vi "averager.vi"() -> ()   [LabVIEW 2015]
uses:
  <vilib>/rvi/IPIntegrationNode/IPINode_Typedef/niFpgaIPINodeSupportedFamilies.ctl
  <vilib>/rvi/Emulation/niFpgaGetClockAttributes.vi
  <vilib>/rvi/Emulation/niFpgaSctlEmulationGetInTimedLoop.vi
  <vilib>/rvi/Emulation/niFpgaEmulationReportErrorSimple.vi
  <vilib>/rvi/IPIntegrationNode/IPINode_Utilities/niFpgaIPINodeSimCore.vi
  <vilib>/rvi/Emulation/niFpgaCriticalErrorInLSC.vi
  <vilib>/rvi/XilinxIP/XIPIN_XNode/niFpgaXIPIN.xnode
  averager/Accumulator/Accumulator_53DC2439CD9149F49F85B82DAD68175F.dll
  <vilib>/rvi/IPIntegrationNode/IPINode_Xnode/niFpgaIPINode.xnode
panel:
  out "Numeric 2":fxp<+/-,32,16>
  out "Numeric":u64
  in  "bypass":bool
  in  "c_in":bool
  in  "Array":fxp<+,32,32>[](array[numeric])
  in  "n":i32
  out "q":bool[](array[boolean])
  in  "sclr":bool
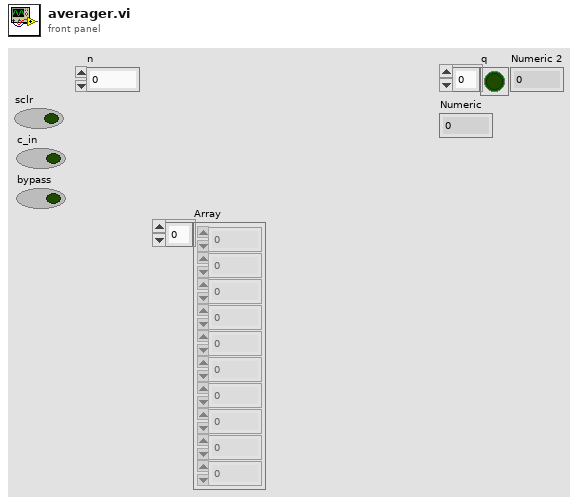
[diagram p1: front panel]
types:
  T1 = typedef "niFpgaIPINodeSupportedFamilies.ctl" = cluster{"unlimited?":bool, "supported targets":string[]}
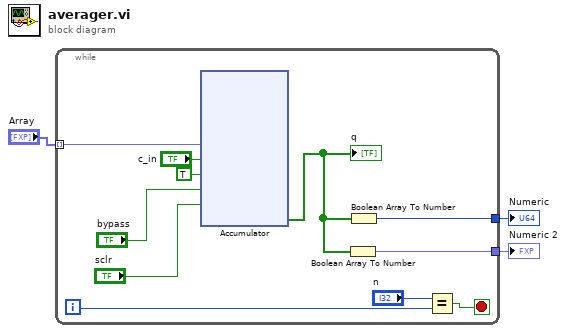
[diagram p0: block diagram]
diagram:
  n1 = while {
    tunnel: "Array" -> [w7] mode=indexing
    tunnel: [w6] -> w1
    tunnel: [w4] -> w2
    i -> [w12]
    stop <- w13 stop-if-true
    n2 = xnode ("Accumulator")("b"=w7, "c_in"="c_in", "ce"=TRUE, "bypass"="bypass", "sclr"="sclr") -> ("q"=w5:bool[])
    "q" <- w5
    n3 = Boolean Array To Number(Boolean array=w5) -> (number=w6:fxp<+/-,32,16>)
    n4 = Boolean Array To Number(Boolean array=w5) -> (number=w4:u64)
    n5 = Equal?(x="n", y=w12) -> (x = y?=w13:bool)
  }
  "Numeric" <- w2
  "Numeric 2" <- w1
